vi "Teleop.vi"(10 "Match Info":T1={"Autonomous Elapsed Seconds"=0.0, "TeleOp Elapsed Seconds"=0.0, "Disabled Elapsed Seconds"=0.0, "Visited Autonomous"=FALSE, "Visited TeleOp"=FALSE, "Visited Disabled"=FALSE, "Autonomous Settings"={"Autonomous Style"=enum."Independent", "VI Refnum"=refnum}}, 11 "Call Context":T2) -> ()   [LabVIEW 2012]
doc: "This VI is called for each TeleOp packet received from the DS where the robot is not disabled. It is often used to read from the joysticks and update I/O or to update setpoints for timed control loops. It should complete and return within 20 milliseconds or it may miss DS packets."
uses:
  <vilib>/Rock Robotics/WPI/DriverStation/WPI_DriverStationDerivedRobotMode.ctl
  <vilib>/Rock Robotics/WPI/DriverStation/WPI_DriverStationMatch Info.ctl
  Robot Global Data.vi
  <vilib>/Rock Robotics/WPI/Joystick/WPI_JoystickGetSetRefNum.vi
panel:
  out "Numeric 1":dbl(slide) scale=0.0..100.0
  out "Boolean 2":bool
  out "Boolean 1":bool
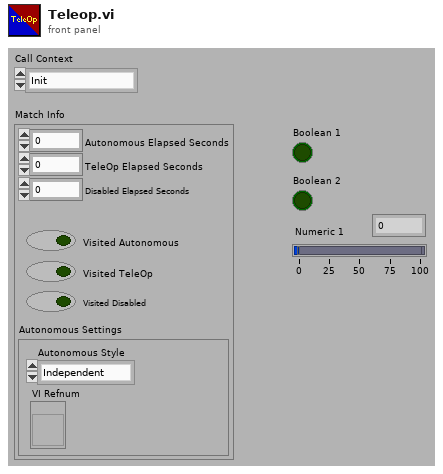
[diagram p1: front panel]
types:
  T1 = typedef "WPI_DriverStationMatch Info.ctl" = cluster{"Autonomous Elapsed Seconds":dbl, "TeleOp Elapsed Seconds":dbl, "Disabled Elapsed Seconds":dbl, "Visited Autonomous":bool, "Visited TeleOp":bool, "Visited Disabled":bool, "Autonomous Settings":cluster{"Autonomous Style":enum16{"Iterative", "Independent"}, "VI Refnum":refnum<vi>}}
  T2 = typedef "WPI_DriverStationDerivedRobotMode.ctl" = enum16{"Init", "Execute", "Stop"}
  T3 = typedef "WPI_RobotDriveDevRef.ctl" = cluster{"DevStatus":errorcluster, "Motors[]":T4[], "Square Inputs":bool, "Max Output":dbl, "Isochronous":bool}
  T4 = typedef "WPI_MotorControlDeviceRef.ctl" = cluster{"DeviceStatus":errorcluster, "Type":enum16{"PWM", "CAN"}, "PWM":cluster{"Digital Module":T5, "PWM Channel":T6, "DeadBand":T7}, "CAN":cluster{"Device Number":u8, "Control Mode":T8, "Semaphore":T9, "Max Vout":dbl}, "Invert":bool, "TransformRef":T10, "InvTransformRef":T10}
  T5 = typedef "FPGA_TypedefDigitalModule.ctl" = enum16{"Digital Module 1", "Digital Module 2"}
  T6 = typedef "FPGA_DIOPWMChannel.ctl" = enum8{"PWM 1", "PWM 2", "PWM 3", "PWM 4", "PWM 5", "PWM 6", "PWM 7", "PWM 8", "PWM 9", "PWM 10", "Invalid"}
  T7 = typedef "WPI_PWMDeadband.ctl" = cluster{"Name":string, "maxPositivePwm":i32, "minPositivePwm":i32, "centerPwm":i32, "maxNegativePwm":i32, "minNegativePwm":i32, "angularRange":u16}
  T8 = typedef "WPI_CANJaguar_ControlMode.ctl" = enum8{"Percent VBus", "Current", "Speed", "Position", "Voltage"}
  T9 = typedef "Semaphore RefNum" = refnum<k1>
  T10 = typedef "WPI_PWMTransform_ConPane.ctl" = refnum<vi>
  T11 = typedef "WPI_JoystickDevRef.ctl" = cluster{"Device":T12}
  T12 = typedef "WPI_JoystickDeviceEnum.ctl" = enum16{"USB 1", "USB 2", "USB 3", "USB 4", "Kinect 1", "Kinect 2"}
  T13 = typedef "WPI_JoystickButtonState.ctl" = cluster{"Button 1":bool, "Button 2":bool, "Button 3":bool, "Button 4":bool, "Button 5":bool, "Button 6":bool, "Button 7":bool, "Button 8":bool, "Button 9":bool, "Button 10":bool, "Button 11":bool, "Button 12":bool}
  T14 = cluster{"axis 1 (x)":dbl, "axis 2 (y)":dbl, "axis 3 (throttle)":dbl, "axis 4":dbl, "axis 5":dbl, "axis 6":dbl}
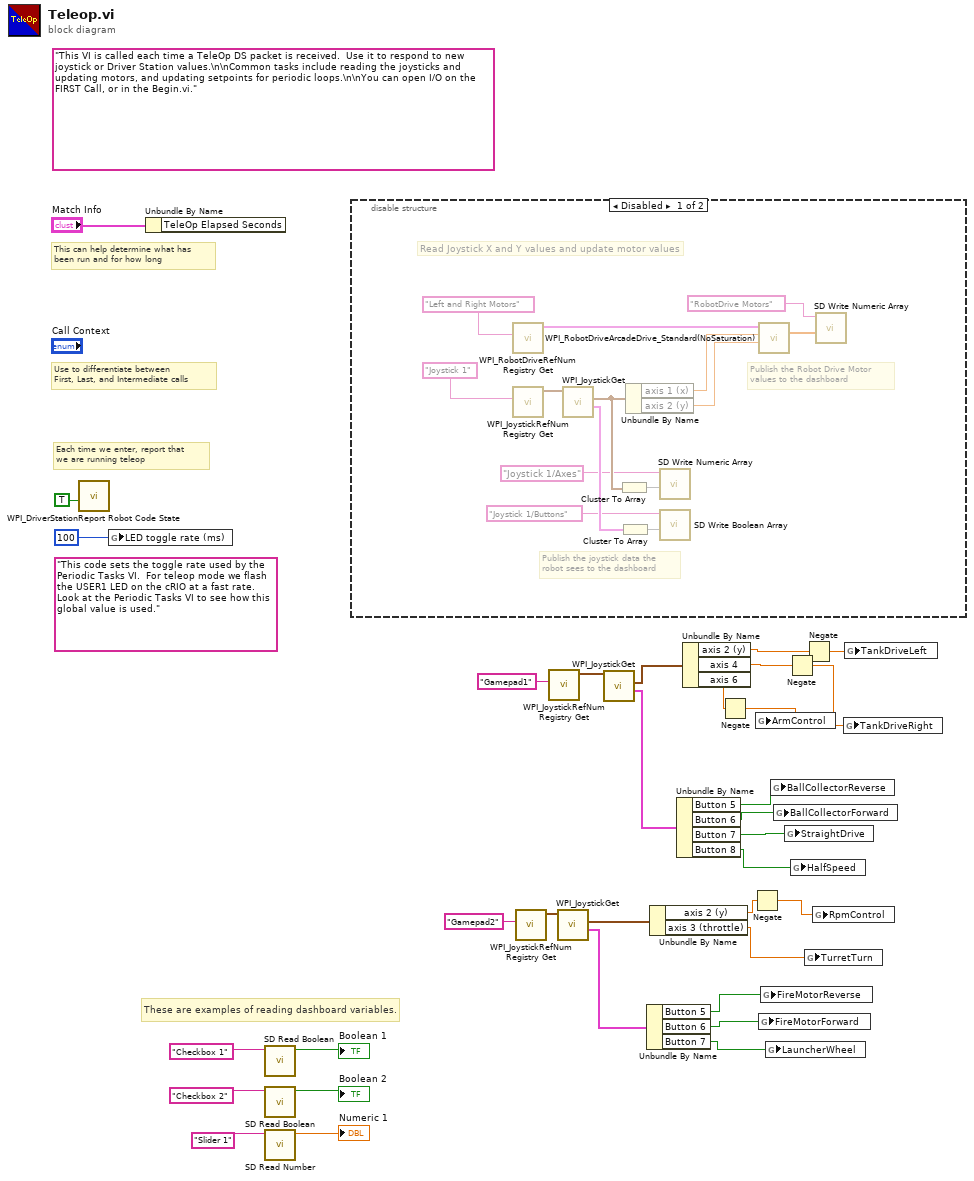
[diagram p0: block diagram]
diagram:
  (unwired) "This code sets the toggle rate used by the Periodic Tasks VI.  For teleop mode we flash the USER1 LED on the cRIO at a fast rate.  Look at the Periodic Tasks VI to see how this global value is used."
  (unwired) "This VI is called each time a TeleOp DS packet is received.  Use it to respond to new joystick or Driver Station values.\n\nCommon tasks include reading the joysticks and updating motors, and updating setpoints for periodic loops.\n\nYou can open I/O on the FIRST Call, or in the Begin.vi."
  # "These are examples of reading dashboard variables."
  # "Each time we enter, report that\nwe are running teleop"
  # "Use to differentiate between\nFirst, Last, and Intermediate calls"
  # "This can help determine what has\nbeen run and for how long"
  n1 = call <vilib>:"WPI_DriverStationReport Robot Code State.vi"("TeleOp"=TRUE ("Autonomous")) -> ()  [unwired: 10 in, 1 out]
  n2 = global write "Robot Global Data.vi" "LED toggle rate (ms)"(u32 100 ("LED ms toggle rate")) -> ()
  n3 = Unbundle By Name("Match Info") -> ()  [unwired: 1 out]
  n4 = call <vilib>:"SD Read Boolean.vi"("Name"="Checkbox 1" ("refnum name")) -> ("Boolean"=→"Boolean 1":bool)  [unwired: 8 in, 2 out]
  n5 = call <vilib>:"SD Read Boolean.vi"("Name"="Checkbox 2" ("refnum name")) -> ("Boolean"=→"Boolean 2":bool)  [unwired: 8 in, 2 out]
  n6 = call <vilib>:"SD Read Number.vi"("Name"="Slider 1" ("refnum name")) -> ("Numeric"=→"Numeric 1":dbl)  [unwired: 8 in, 2 out]
  n7 = disable-structure shown="Disabled" {
    frame Disabled {
      # "Publish the Robot Drive Motor\nvalues to the dashboard"
      # "Publish the joystick data the\nrobot sees to the dashboard"
      # "Read Joystick X and Y values and update motor values"
      n8 = call <vilib>:"WPI_RobotDriveRefNum Registry Get.vi"("refnum name"="Left and Right Motors") -> ("RobotDriveDevRef"=w46:T3)  [unwired: 1 in, 9 out]
      n9 = call <vilib>:"WPI_JoystickRefNum Registry Get.vi"("refnum name"="Joystick 1") -> ("JoystickDevRef"=w42:T11)  [unwired: 1 in, 9 out]
      n10 = call <vilib>:"WPI_JoystickGet.vi"("JoystickDevRef"=w42) -> ("Buttons"=w41:T13, "Axes"=w38:T14)  [unwired: 1 in, 4 out]
      n11 = Cluster To Array(cluster=w38) -> (array=w37:dbl[])
      n12 = Cluster To Array(cluster=w41) -> (array=w40:bool[])
      n13 = Unbundle By Name(w38) -> ("axis 1 (x)"=w45:dbl, "axis 2 (y)"=w44:dbl)
      n14 = call <vilib>:"SD Write Numeric Array.vi"("Numeric Array"=w37, "Name"="Joystick 1/Axes") -> ()  [unwired: 8 in, 2 out]
      n15 = call <vilib>:"SD Write Boolean Array.vi"("Boolean Array"=w40, "Name"="Joystick 1/Buttons") -> ()  [unwired: 8 in, 2 out]
      n16 = call <vilib>:"WPI_RobotDriveArcadeDrive_Standard(NoSaturation).vi"("Y axis value"=w44, "X axis value"=w45, "RobotDriveDevRef"=w46) -> ("Motor Values"=w34:dbl[])  [unwired: 1 in, 7 out]
      n17 = call <vilib>:"SD Write Numeric Array.vi"("Numeric Array"=w34, "Name"="RobotDrive Motors") -> ()  [unwired: 8 in, 2 out]
    }
    frame Enabled {
    }
  }
  n18 = call <vilib>:"WPI_JoystickRefNum Registry Get.vi"("refnum name"="Gamepad2") -> ("JoystickDevRef"=w21:T11)  [unwired: 1 in, 9 out]
  n19 = call <vilib>:"WPI_JoystickRefNum Registry Get.vi"("refnum name"="Gamepad1") -> ("JoystickDevRef"=w22:T11)  [unwired: 1 in, 9 out]
  n20 = call <vilib>:"WPI_JoystickGet.vi"("JoystickDevRef"=w21) -> ("Buttons"=w11:T13, "Axes"=w6:T14)  [unwired: 4 in, 1 out]
  n21 = call <vilib>:"WPI_JoystickGet.vi"("JoystickDevRef"=w22) -> ("Buttons"=w19:T13, "Axes"=w20:T14)  [unwired: 4 in, 1 out]
  n22 = Unbundle By Name(w11) -> ("Button 5"=w2:bool, "Button 6"=w1:bool, "Button 7"=w10:bool)
  n23 = Unbundle By Name(w6) -> ("axis 2 (y)"=w8:dbl, "axis 3 (throttle)"=w3:dbl)
  n24 = Unbundle By Name(w19) -> ("Button 5"=w15:bool, "Button 6"=w12:bool, "Button 7"=w14:bool, "Button 8"=w13:bool)
  n25 = Unbundle By Name(w20) -> ("axis 2 (y)"=w18:dbl, "axis 4"=w17:dbl, "axis 6"=w5:dbl)
  n26 = Negate(x=w5) -> (-x=w4:dbl)
  n27 = Negate(x=w8) -> (-x=w7:dbl)
  n28 = global write "Robot Global Data.vi" "ArmControl"(w4) -> ()
  n29 = global write "Robot Global Data.vi" "FireMotorForward"(w1) -> ()
  n30 = global write "Robot Global Data.vi" "FireMotorReverse"(w2) -> ()
  n31 = global write "Robot Global Data.vi" "LauncherWheel"(w10) -> ()
  n32 = global write "Robot Global Data.vi" "BallCollectorReverse"(w15) -> ()
  n33 = global write "Robot Global Data.vi" "BallCollectorForward"(w12) -> ()
  n34 = global write "Robot Global Data.vi" "StraightDrive"(w14) -> ()
  n35 = Negate(x=w17) -> (-x=w16:dbl)
  n36 = global write "Robot Global Data.vi" "HalfSpeed"(w13) -> ()
  n37 = Negate(x=w18) -> (-x=w9:dbl)
  n38 = global write "Robot Global Data.vi" "TurretTurn"(w3) -> ()
  n39 = global write "Robot Global Data.vi" "RpmControl"(w7) -> ()
  n40 = global write "Robot Global Data.vi" "TankDriveRight"(w16) -> ()
  n41 = global write "Robot Global Data.vi" "TankDriveLeft"(w9) -> ()
